vi "Ball-Detect(Color).vi"() -> (7 "See":bool)   [LabVIEW 2019]
uses:
  Robot Global Data.vi
  <vilib>/Rock Robotics/SystemInterfaces/i2clib/i2c_bus.ctl
panel:
  in  "Other":cluster{"R":dbl, "G":dbl, "B":dbl}={"R"=0.361, "G"=0.524, "B"=0.113}
  in  "Blue Calibration":cluster{"R":dbl, "G":dbl, "B":dbl}={"R"=0.143, "G"=0.427, "B"=0.429}
  in  "Green Calibration":cluster{"R":dbl, "G":dbl, "B":dbl}={"R"=0.197, "G"=0.561, "B"=0.24}
  in  "Red Calibration":cluster{"R":dbl, "G":dbl, "B":dbl}={"R"=0.561, "G"=0.323, "B"=0.114}
  in  "Yellow Calibration":cluster{"R":dbl, "G":dbl, "B":dbl}={"R"=0.361, "G"=0.524, "B"=0.113}
  in  "I2C Bus":T1
  out "Color":u32(colorbox)
  out "Proximity":u16(graph)
  out "error out":errorcluster
  out "Measured Color":cluster{"R":dbl, "G":dbl, "B":dbl}
  out "Match Confidence":dbl
  out "Matched Color Name":string
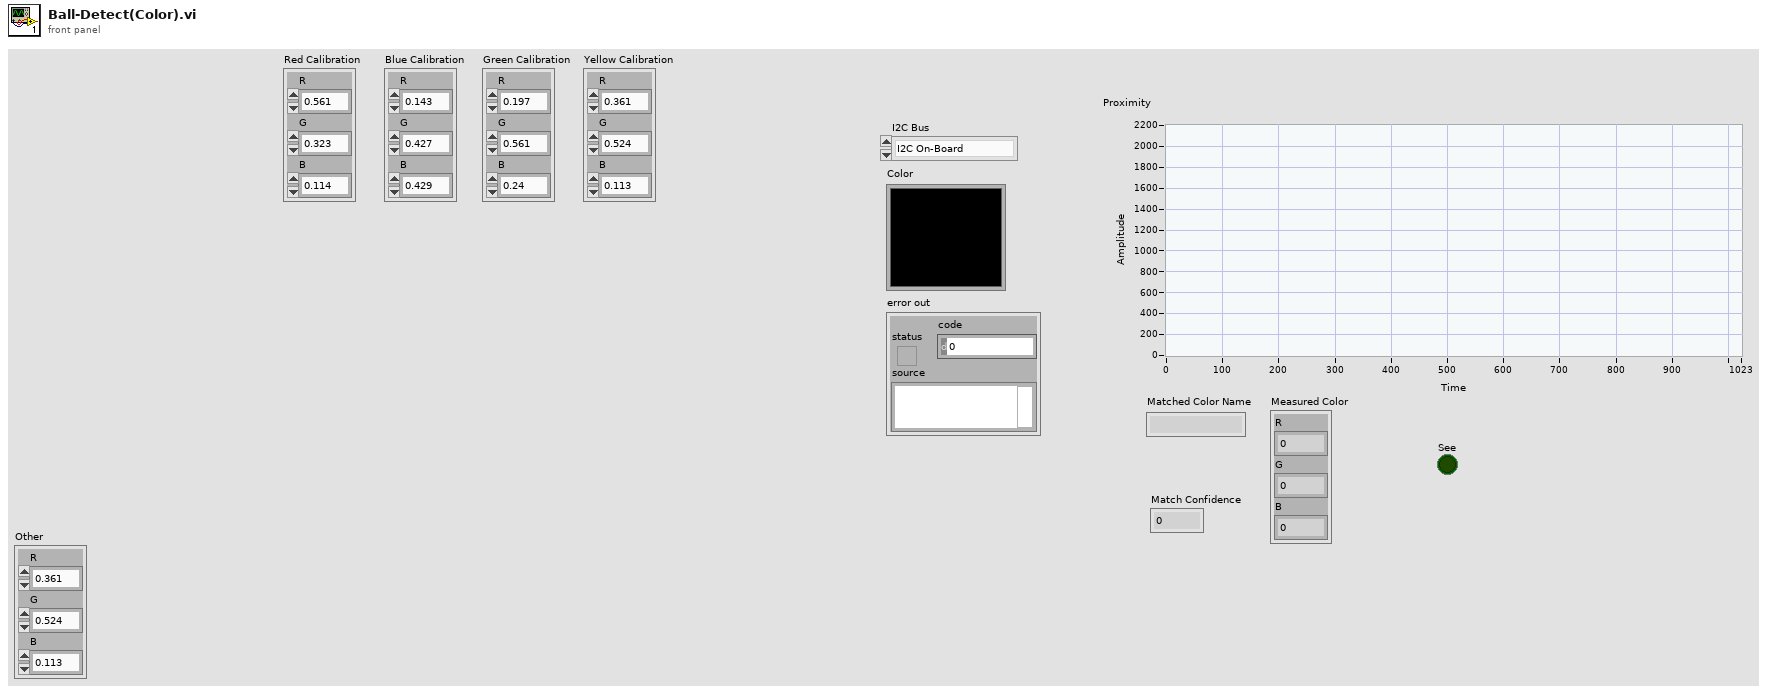
[diagram p1: front panel]
types:
  T1 = typedef "i2c_bus.ctl" = enum16{"I2C On-Board", "I2C MXP", "Invalid"}
  T2 = typedef "Color Sensor V3 DevRef.ctl" = cluster{"I2CDevRef":T3}
  T3 = typedef "WPI_I2CDevRef.ctl" = cluster{"DevStatus":errorcluster, "Device Address":u8, "Handle":i32, "I2C Bus":T1}
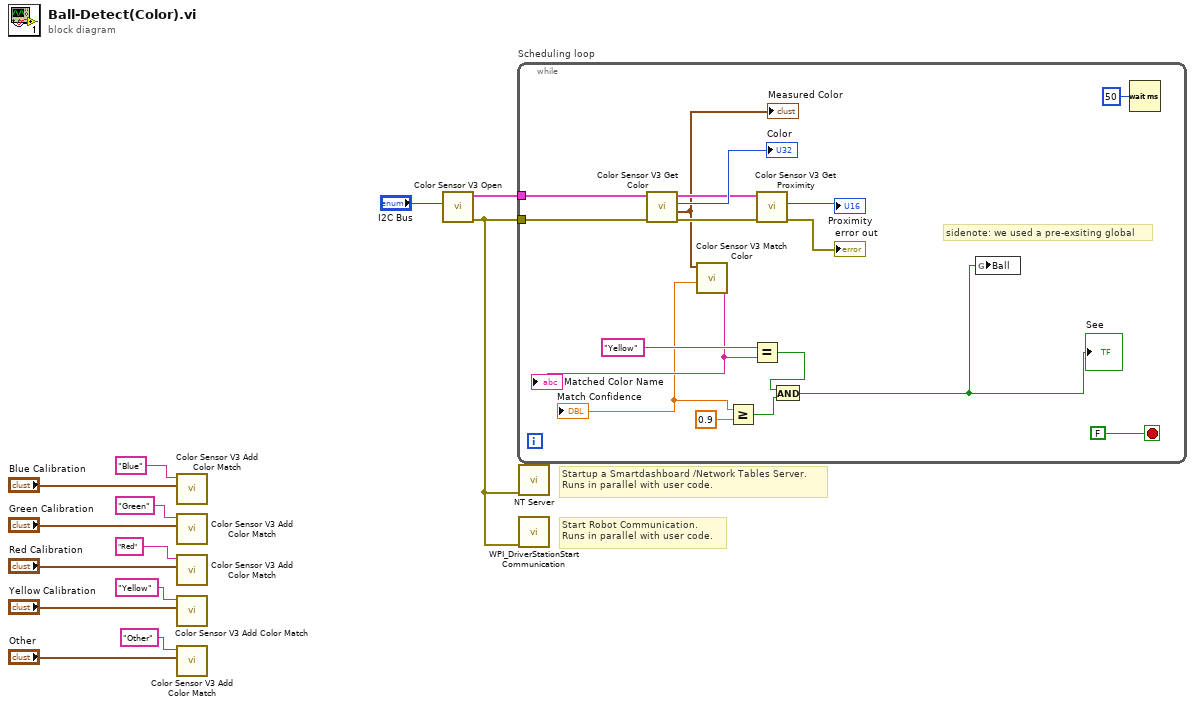
[diagram p0: block diagram]
diagram:
  # "Startup a Smartdashboard /Network Tables Server.\nRuns in parallel with user code."
  # "Start Robot Communication.\nRuns in parallel with user code."
  n1 = call <vilib>:"Color Sensor V3 Add Color Match.vi"("Color"="Blue Calibration", "Name"="Blue") -> ()  [unwired: 10 in]
  n2 = call <vilib>:"Color Sensor V3 Add Color Match.vi"("Color"="Green Calibration", "Name"="Green") -> ()  [unwired: 10 in]
  n3 = call <vilib>:"Color Sensor V3 Add Color Match.vi"("Color"="Red Calibration", "Name"="Red") -> ()  [unwired: 10 in]
  n4 = call <vilib>:"Color Sensor V3 Add Color Match.vi"("Color"="Yellow Calibration", "Name"="Yellow") -> ()  [unwired: 10 in]
  n5 = call <vilib>:"Color Sensor V3 Add Color Match.vi"("Color"="Other", "Name"="Other") -> ()  [unwired: 10 in]
  n6 = call <vilib>:"Color Sensor V3 Open.vi"("I2C Bus"="I2C Bus") -> ("error out"=w11:errorcluster, "ColorSensorDevRef"=w12:T2)  [unwired: 9 in]
  n7 = while "Scheduling loop" {
    tunnel: w12 -> [w24]
    tunnel: w11 -> [w23]
    stop <- FALSE stop-if-true
    # "sidenote: we used a pre-exsiting global"
    n8 = call <vilib>:"Color Sensor V3 Get Color.vi"("error in (no error)"=w23, "ColorSensorDevRef"=w24) -> ("error out"=w28:errorcluster, "Normalized Color"=w22:cluster{"R":dbl, "G":dbl, "B":dbl}, "Color"=→"Color":u32, "ColorSensorDevRef out"=w27:T2)  [unwired: 6 in]
    "Measured Color" <- w22
    n9 = call <vilib>:"Color Sensor V3 Match Color.vi"("Measured Color"=w22) -> ("Confidence"=w18:dbl, "Matched Color Name"=w19:string)  [unwired: 8 in, 1 out]
    "Match Confidence" <- w18
    "Matched Color Name" <- w19
    n10 = Greater Or Equal?(x=w18, y=0.9) -> (x >= y?=w16:bool)
    n11 = Equal?(x="Yellow", y=w19) -> (x = y?=w15:bool)
    n12 = call <vilib>:"Color Sensor V3 Get Proximity.vi"("error in (no error)"=w28, "ColorSensorDevRef"=w27) -> ("error out"=→"error out":errorcluster, "Proximity"=→"Proximity":u16)  [unwired: 7 in, 1 out]
    n13 = And(x=w15, y=w16) -> (x .and. y?=w14:bool)
    "See" <- w14
    n14 = global write "Robot Global Data.vi" "Ball"(w14) -> ()
    n15 = Wait (ms)(milliseconds to wait=u32 50) -> ()  [unwired: 1 out]
  }
  n16 = call <vilib>:"NT Server.vi"("error in (no error)"=w11) -> ()  [unwired: 11 in]
  n17 = call <vilib>:"WPI_DriverStationStart Communication.vi"("error in (no error)"=w11) -> ()  [unwired: 1 in, 10 out]
